vi "green buoy2.0.vi"(7 "error in (no error)":errorcluster, 8 "Cluster":cluster{"Max Radius":sgl, "Min Radius":sgl}={"Max Radius"=50.0, "Min Radius"=9.0}, 10 "Image Src":T2) -> (0 "error out":errorcluster, 1 "Nb Circles":i32, 2 "Circles Data (calibrated)":T1(array[cluster]), 3 "Image Out":T2(plugin-control))   [LabVIEW 2009]
uses:
  <vilib>/vision/Image Controls.llb/IMAQ Image.ctl
  <vilib>/vision/NI_Vision_Development_Module.lvlib
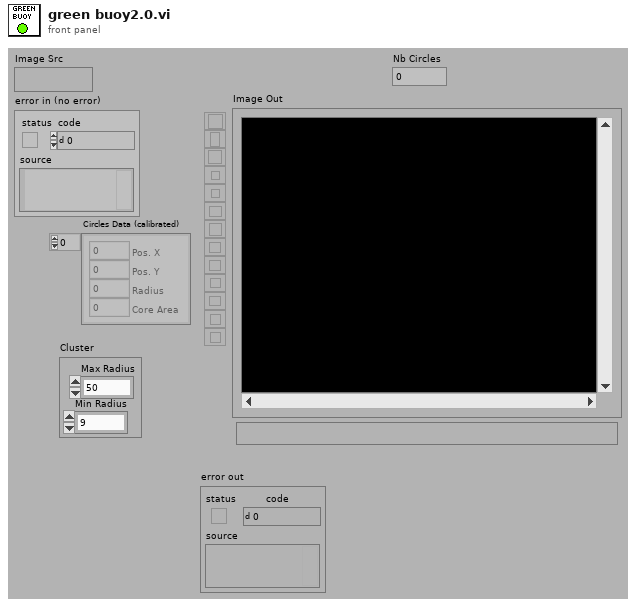
[diagram p1: front panel]
types:
  T1 = cluster{"Pos. X":i32, "Pos. Y":i32, "Radius":i32, "Core Area":i32}[]
  T2 = typedef "IMAQ Image.ctl" = refnum<image>
  T3 = enum32{"AutoM", "Close", "Dilate", "Erode", "Gradient", "Gradient out", "Gradient in", "Hit miss", "Open", "PClose", "POpen", "Thick", "Thin"}
  T4 = enum32{"AutoM", "Close", "Dilate", "Erode", "Gradient", "Gradient in", "Gradient out", "HitMiss", "Open", "PClose", "POpen", "Thick", "Thin"}
  T5 = enum32{"Linear", "Log", "Exp", "Square", "Square root", "Power X", "Power 1/X"}
  T6 = cluster{"Brightness":sgl, "Contrast":sgl, "Gamma":sgl}
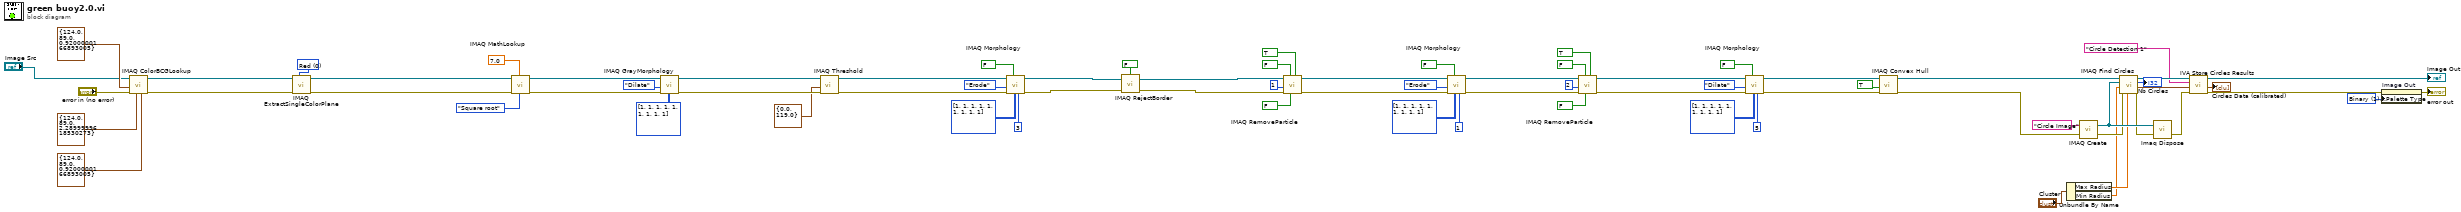
[diagram p0: block diagram]
diagram:
  w9 = u32 1 items=["Grayscale", "Binary", "Gradient", "Rainbow", "Temperature", "User Defined"] ("Palette")
  w69 = 0 items=["Red", "Green", "Blue", "Hue", "Saturation", "Luminance", "Value", "Intensity"] ("Color Plane")
  n1 = call "IMAQ ColorBCGLookup"("Blue BCG Values"=T6 {"Brightness"=124.0, "Contrast"=89.0, "Gamma"=0.92}, "Green BCG Values"=T6 {"Brightness"=124.0, "Contrast"=89.0, "Gamma"=2.29}, "error in (no error)"="error in (no error)", "Red BCG Values"=T6 {"Brightness"=124.0, "Contrast"=89.0, "Gamma"=0.92}, "Image Src"="Image Src") -> ("error out"=w73:errorcluster, "Image Dst Out"=w68:T2)  [unwired: 2 in, 3 out]
  n2 = call "IMAQ ExtractSingleColorPlane"("Color Plane"=w69, "error in (no error)"=w73, "Image Src"=w68) -> ("error out"=w67:errorcluster, "Image Dst Out"=w64:T2)  [unwired: 1 in, 6 out]
  n3 = call "IMAQ MathLookup"("Operator"=T5."Square root", "X Value"=sgl 7.0, "error in (no error)"=w67, "Image Src"=w64) -> ("error out"=w63:errorcluster, "Image Dst Out"=w60:T2)  [unwired: 3 in, 3 out]
  n4 = call "IMAQ GrayMorphology"("Structuring Element"=i32[][] [[1, 1, 1], [1, 1, 1], [1, 1, 1]], "error in (no error)"=w63, "Operation"=T4."Dilate", "Image Src"=w60) -> ("error out"=w59:errorcluster, "Image Dst Out"=w57:T2)  [unwired: 3 in, 3 out]
  n5 = call "IMAQ Threshold"("error in (no error)"=w59, "Range"=cluster{"Lower value":sgl, "Upper value":sgl} {"Lower value"=0.0, "Upper value"=119.0}, "Image Src"=w57) -> ("error out"=w56:errorcluster, "Image Dst Out"=w51:T2)  [unwired: 3 in, 4 out]
  n6 = call "IMAQ Morphology"("Number of iterations (1)"=3, "Structuring Element"=i32[][] [[1, 1, 1], [1, 1, 1], [1, 1, 1]], "Square/Hexa (Square)"=FALSE, "error in (no error)"=w56, "Operation"=T3."Erode", "Image Src"=w51) -> ("error out"=w50:errorcluster, "Image Dst Out"=w48:T2)  [unwired: 1 in, 3 out]
  n7 = call "IMAQ RejectBorder"("error in (no error)"=w50, "Image Src"=w48, "Connectivity 4/8 (8)"=FALSE) -> ("error out"=w47:errorcluster, "Image Dst Out"=w42:T2)  [unwired: 1 in, 2 out]
  n8 = call "IMAQ RemoveParticle"("Connectivity 4/8 (8)"=TRUE, "Low Pass/High Pass (Low)"=FALSE, "Square/Hexa (Square)"=FALSE, "error in (no error)"=w47, "Number of Erosion"=1, "Image Src"=w42) -> ("error out"=w41:errorcluster, "Image Dst Out"=w36:T2)  [unwired: 1 in, 3 out]
  n9 = call "IMAQ Morphology"("Number of iterations (1)"=1, "Structuring Element"=i32[][] [[1, 1, 1], [1, 1, 1], [1, 1, 1]], "Square/Hexa (Square)"=FALSE, "error in (no error)"=w41, "Operation"=T3."Erode", "Image Src"=w36) -> ("error out"=w35:errorcluster, "Image Dst Out"=w30:T2)  [unwired: 1 in, 3 out]
  n10 = call "IMAQ RemoveParticle"("Connectivity 4/8 (8)"=TRUE, "Low Pass/High Pass (Low)"=FALSE, "Square/Hexa (Square)"=FALSE, "error in (no error)"=w35, "Number of Erosion"=2, "Image Src"=w30) -> ("error out"=w29:errorcluster, "Image Dst Out"=w24:T2)  [unwired: 1 in, 3 out]
  n11 = call "IMAQ Morphology"("Number of iterations (1)"=5, "Structuring Element"=i32[][] [[1, 1, 1], [1, 1, 1], [1, 1, 1]], "Square/Hexa (Square)"=FALSE, "error in (no error)"=w29, "Operation"=T3."Dilate", "Image Src"=w24) -> ("error out"=w23:errorcluster, "Image Dst Out"=w22:T2)  [unwired: 1 in, 3 out]
  n12 = call "IMAQ Convex Hull"("error in (no error)"=w23, "Connectivity 4/8 (8)"=TRUE, "Image Src"=w22) -> ("error out"=w20:errorcluster, "Image Dst Out"=w13:T2)  [unwired: 1 in, 6 out]
  n13 = Unbundle By Name("Cluster") -> ("Max Radius"=w2:sgl, "Min Radius"=w1:sgl)
  n14 = call "IMAQ Create"("Image Name"="Circle Image", "error in (no error)"=w20) -> ("New Image"=w18:T2, "error out"=w17:errorcluster)  [unwired: 2 in, 1 out]
  n15 = call "IMAQ Find Circles"("Max Radius"=w2, "error in (no error)"=w17, "Min Radius"=w1, "Image Dst"=w18, "Image Src"=w13) -> ("error out"=w16:errorcluster, "Circles Data"=w11:T1, "Nb Circles"=→"Nb Circles":i32)  [unwired: 4 out]
  n16 = call "Imaq Dispose"("Image"=w18, "error in (no error)"=w16) -> ("error out"=w15:errorcluster)  [unwired: 1 in, 3 out]
  n17 = call <vilib>:"IVA Store Circles Results.vi"("error in (no error)"=w15, "Circles Data"=w11, "Step Name"="Circle Detection 1", "Image in"=w13) -> ("error out"=w14:errorcluster, "Circles Data (calibrated)"=→"Circles Data (calibrated)":T1, "Image dup"=→"Image Out":T2)  [unwired: 5 out]
  n18 = property on="Image Out" class="ImageControl"(error in=w14, "Palette:Palette Type"=w9) -> (error out=→"error out":errorcluster)  [unwired: 1 in, 1 out]
